vi "Activity log controller.vi"(0 "Mode":T4(ring), 1 "Activity log filepath":path, 5 "Max seconds between DITs":dbl=28800.0, 7 "Bypass activities? (F)":bool, 9 "New activities":T2 {"Epoch sec" format="%.2e"}, 11 "error in (no error)":errorcluster, 12 "DIT Key Info":T1) -> (15 "error out":errorcluster)   [LabVIEW 2012]
doc: "This vi handles all write operations to an activity log at \"activity log filepath\". It is called in one of 5 modes:\n\n1)Initialize: Checks if the activity log exists. If it doesn't creates and adds first row with creation date. If the log exists, checks if there is any text at the end of the file that is not followed by a DIT. If there is, a special <DIT></DIT> seperator is added to the file.\n\n2)Write activities to file: Appends 1 or more lines to the log (1 for each entry in the input \"new activities\" array) with date/time and activity. Doesn't add DIT to file. Keeps track of the text added to the file for later adding of DIT.\n\n3) Write DIT: writes a DIT tag to the end of the file based on text that has been added but that does not have a DIT associated with it.\n\n4) Time to add DIT?: This vi should be called periodically in this mode to check if the time interval since initialization or the last writing of a DIT is greater than \"max seconds between DITs\". If so, a DIT is automatically added to the log, then the timer for this function reset.\n\nIf the input \"Bypass activities?\" = T, this vi does nothing."
uses:
  User Access Type defs/Acitivity cluster array.ctl
  User Access Type defs/Acitivity cluster.ctl
  User Access Type defs/DIT Key cluster.ctl
panel:
  # "for write only"
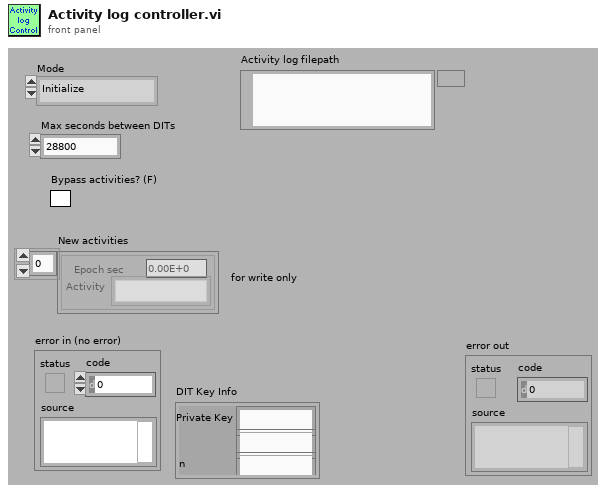
[diagram p1: front panel]
types:
  T1 = typedef "DIT Key cluster.ctl" = cluster{"Private Key":string, "Public Key":string, "n":string}
  T2 = typedef "Acitivity cluster array.ctl" = T3[]
  T3 = typedef "Acitivity cluster.ctl" = cluster{"Epoch sec":dbl, "Activity":string}
  T4 = enum16{"Initialize", "Write activities to file", "Write DIT", "Time to add DIT?"}
  T5 = enum16{"Initialize", "Write activities to file", "Write to file with DIT", "Time to add DIT?", "Add DIT"}
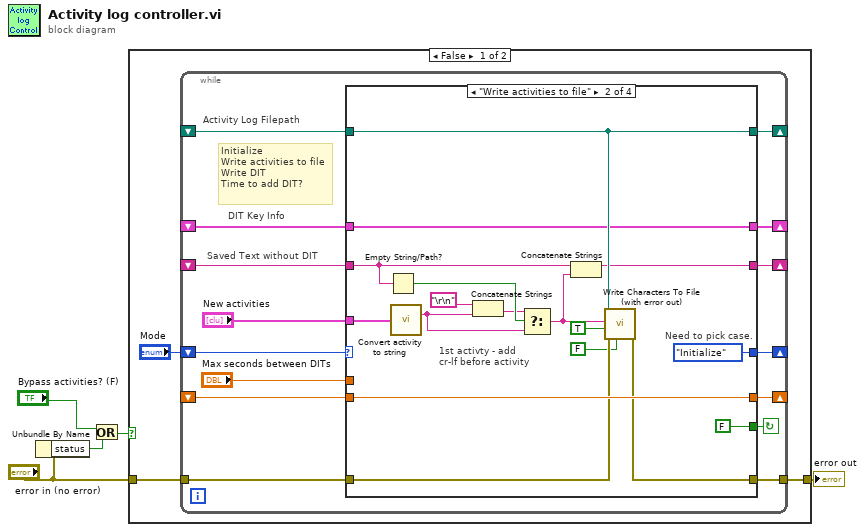
[diagram p0: block diagram]
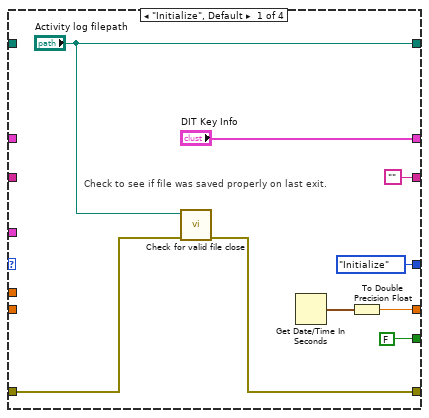
[diagram p2: hidden frame]
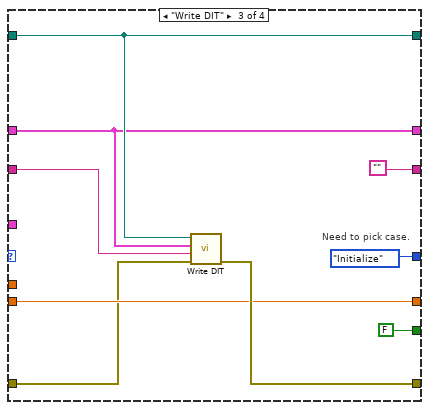
[diagram p3: hidden frame]
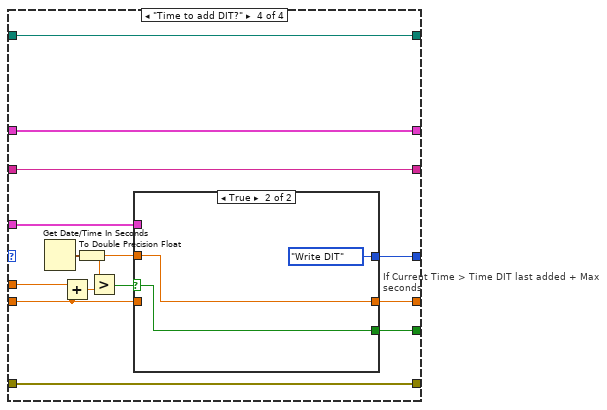
[diagram p4: hidden frame]
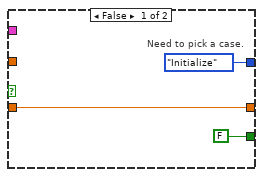
[diagram p5: hidden frame]
diagram:
  n1 = Unbundle By Name("error in (no error)") -> ("status"=w3:bool)
  n2 = Or(x="Bypass activities? (F)", y=w3) -> (x .or. y?=w1:bool)
  n3 = case shown="False" w1 {
    tunnel: [w8 w79] -> w5
    tunnel: "error in (no error)" -> [w6 w79]
    frame False {
      n4 = while {
        tunnel: w6 -> [w18]
        tunnel: [w22] -> w8
        shift-right: [w20] -> _
        shift-left: _ -> [w19]
        shift-right: [w15] -> _
        shift-left: "Mode" -> [w17]
        shift-right: [w11] -> _
        shift-left: _ -> [w12]
        shift-right: [w13] -> _
        shift-left: _ -> [w14]
        shift-right: [w10] -> _
        shift-left: _ -> [w9]
        stop <- w16 continue-if-true
        # "Initialize\nWrite activities to file\nWrite DIT\nTime to add DIT?"
        # "DIT Key Info"
        # "Activity Log Filepath"
        # "Saved Text without DIT"
        n5 = case shown="\"Write activities to file\"" w17 {
          tunnel: "New activities" -> [_ w43 _ w65]
          tunnel: w18 -> [w26 w47 w54 w72]
          tunnel: [w25 w46 w58 w72] -> w22
          tunnel: "Max seconds between DITs" -> [_ _ _ w71]
          tunnel: [w32 w49 w57 w67] -> w20
          tunnel: w19 -> [_ w49 w57 w68]
          tunnel: [FALSE FALSE FALSE w64] -> w16
          tunnel: [T4."Initialize" ("Mode") T4."Initialize" ("Mode") T4."Initialize" ("Mode") w63] -> w15
          tunnel: w14 -> [_ w44 w55 w62]
          tunnel: ["Activity log filepath" w44 w55 w62] -> w13
          tunnel: w12 -> [_ w38 w53 w61]
          tunnel: ["" w42 "" w61] -> w11
          tunnel: w9 -> [_ w41 w52 w60]
          tunnel: ["DIT Key Info" w41 w52 w60] -> w10
          frame "Initialize", Default {
            # "Check to see if file was saved properly on last exit."
            n6 = call "Check for valid file close.vi"("error in (no error)"=w26, "Activity log filepath"="Activity log filepath") -> ("error out"=w25:errorcluster)  [unwired: 5 out]
            n7 = Get Date/Time In Seconds() -> (seconds since 1Jan1904=w24:timestamp)
            n8 = To Double Precision Float(number=w24) -> (double precision float=w32:dbl)
          }
          frame "Write activities to file" {
            # "1st activty - add\ncr-lf before activity"
            # "Need to pick case."
            n9 = Empty String/Path?(string/path=w38) -> (empty?=w37:bool)
            n10 = call "Convert activity to string.vi"("Activity log In"=w43) -> ("Activity log string"=w36:string)  [unwired: 4 out]
            n11 = Concatenate Strings("\r\n", w36) -> (w35:string)
            n12 = Select(t=w35, s=w37, f=w36) -> (s? t:f=w34:string)
            n13 = Concatenate Strings(w38, w34) -> (w42:string)
            n14 = call "Write Characters To File (with error out).vi"("advisory dialog? (display:T)"=FALSE, "error in (no error)"=w47, "append to file? (new file:F)"=TRUE, "character string"=w34, "file path (dialog if empty)"=w44) -> ("error out"=w46:errorcluster)  [unwired: 2 in, 4 out]
          }
          frame "Write DIT" {
            # "Need to pick case."
            n15 = call "Write DIT.vi"("error in"=w54, "String"=w53, "DIT Key Info"=w52, "Filepath In"=w55) -> ("error out"=w58:errorcluster)  [unwired: 1 in, 4 out]
          }
          frame "Time to add DIT?" {
            n16 = Get Date/Time In Seconds() -> (seconds since 1Jan1904=w59:timestamp)
            n17 = Add(x=w71, y=w68) -> (x+y=w70:dbl)
            n18 = To Double Precision Float(number=w59) -> (double precision float=w66:dbl)
            n19 = Greater?(x=w66, y=w70) -> (0:w69:bool)
            n20 = case "If Current Time > Time DIT last added + Max seconds" shown="True" w69 {
              selector: w69 -> [_ w77]
              tunnel: w68 -> [w75 _]
              tunnel: [w75 w78] -> w67
              tunnel: w66 -> [_ w78]
              tunnel: w65 -> [_ _]
              tunnel: [FALSE w77] -> w64
              tunnel: [T4."Initialize" ("Mode") T4."Write DIT" ("Mode")] -> w63
              frame False {
                # "Need to pick a case."
              }
              frame True {
                (unwired) T5."Write to file with DIT" ("Mode")
                # "Add DIT to file."
              }
            }
          }
        }
      }
    }
    frame True {
    }
  }
  "error out" <- w5
